vi "Initialize.vi"(0 "Export in":refnum<class "Export.lvclass">) -> (4 "Export out":refnum<class "Export.lvclass">)   [LabVIEW 2017, in "CL_G3_VIComponentBuilder.lvlib" / "Export.lvclass"]
doc: "Responsible for determining the Unique Name, Product Name, and Export's Build Specification file. Initialization involves preforming calculations or actions needed to make the object useable. <RequiredOverrideReason>The way in which the product name, unique name and Export's build spec file is determined is type specific.</RequiredOverrideReason>\n<MustCallParent>The parent preforms the testing to make sure the Unique Name, Product Name, and Export's Build Specification file are correctly set.</MustCallParent>"
uses:
  Export.lvclass
  Export.lvclass/Export.ctl
  Accessors/Read unique Name.vi
  Accessors/Read Product Name.vi
  Accessors/Read Export Build Specification.vi
  Accessors/Write Export Operation Errors.vi
  Accessors/Read Export Operation Errors.vi
  <userlib>/_OpenG.lib/file/file.llb/Valid Path - Traditional__ogtk.vi
  <userlib>/_OpenG.lib/array/array.llb/Search 1D Array (Boolean)__ogtk.vi
  <userlib>/_OpenG.lib/array/array.llb/Index 1D Array Elements (String)__ogtk.vi
  <vilib>/Utility/error.llb/Error Cluster From Error Code.vi
  <vilib>/ErrorRing/Error Ring.xnode
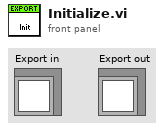
[diagram p1: front panel]
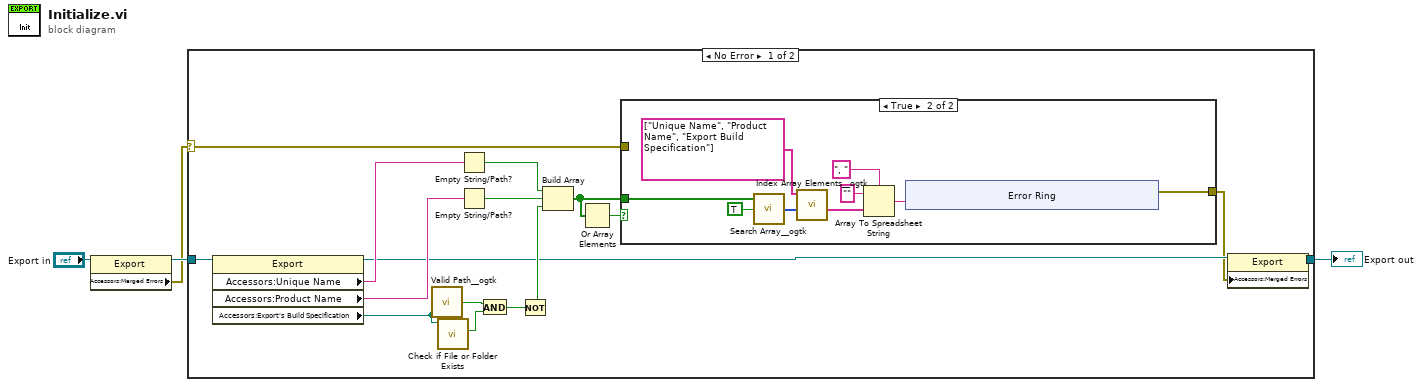
[diagram p0: block diagram]
diagram:
  n1 = property class="Export"(reference="Export in") -> (reference out=w2:refnum<class "Export.lvclass">, "Accessors:Merged Errors"=w1:errorcluster)  [unwired: 1 in, 1 out]
  n2 = case shown="No Error" w1 {
    selector: w1 -> [w17 _]
    tunnel: [w7 w38] -> w4
    tunnel: w2 -> [w5 w38]
    frame No Error {
      n3 = property class="Export"(reference=w5) -> (reference out=w8:refnum<class "Export.lvclass">, "Accessors:Unique Name"=w11:string, "Accessors:Product Name"=w10:string, "Accessors:Export's Build Specification"=w9:path)  [unwired: 1 in, 1 out]
      n4 = call-poly <userlib>:"Valid Path__ogtk.vi"("path"=w9) -> ("valid"=w14:bool)
      n5 = call <vilib>:"Check if File or Folder Exists.vi"("path"=w9) -> ("file or folder exists?"=w13:bool)  [unwired: 8 in, 2 out]
      n6 = Empty String/Path?(string/path=w11) -> (empty?=w20:bool)
      n7 = Empty String/Path?(string/path=w10) -> (empty?=w19:bool)
      n8 = And(x=w14, y=w13) -> (x .and. y?=w12:bool)
      n9 = Not(x=w12) -> (.not. x?=w15:bool)
      n10 = Build Array(w20, w19, w15) -> (w16:bool[])
      n11 = Or Array Elements(Boolean array=w16) -> (logical OR=w18:bool)
      n12 = case shown="True" w18 {
        tunnel: w17 -> [w21 _]
        tunnel: w16 -> [_ w30]
        tunnel: [w21 w22] -> w6
        frame False {
        }
        frame True {
          n13 = call-poly <userlib>:"Search Array__ogtk.vi"("Array"=w30, "Element Data"=TRUE) -> ("Indices of Elements"=w28:i32[])  [unwired: 7 in]
          n14 = call-poly <userlib>:"Index Array Elements__ogtk.vi"("indices"=w28, "array"=string[] ["Unique Name", "Product Name", "Export Build Specification"]) -> ("elements"=w26:string[])  [unwired: 9 in]
          n15 = Array To Spreadsheet String(delimiter (Tab)=", ", array=w26, 3:"" ("format string")) -> (spreadsheet string=w23:string)
          n16 = xnode "Error Ring"("parameter 0"=w23) -> ("error out"=w22:errorcluster)
        }
      }
      n17 = property class="Export"(reference=w8, "Accessors:Merged Errors"=w6) -> (reference out=w7:refnum<class "Export.lvclass">)  [unwired: 1 in, 1 out]
    }
    frame Error {
    }
  }
  "Export out" <- w4
